vi "Calculadora.vi"() -> ()   [LabVIEW 2019, in "Calculadora.lvlib"]
uses:
  Calculadora.lvlib
panel:
  out "Resultado":dbl
  in  "Borrar":bool
  in  "Division":bool
  in  "Multiplicacion":bool
  in  "Resta":bool
  in  "Numero":dbl
  in  "Suma":bool
  # "CALCULADORA"
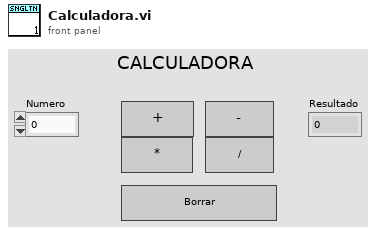
[diagram p1: front panel]
types:
  T1 = typedef "Calculadora.lvlib/Broadcast Events--cluster.ctl" = cluster{"Module Did Init":refnum<user-event>, "Status Updated":refnum<user-event>, "Error Reported":refnum<user-event>, "Did Something":refnum<user-event>, "Module Did Stop":refnum<user-event>, "Update Module Execution Status":refnum<user-event>, "Resultado":refnum<user-event>}
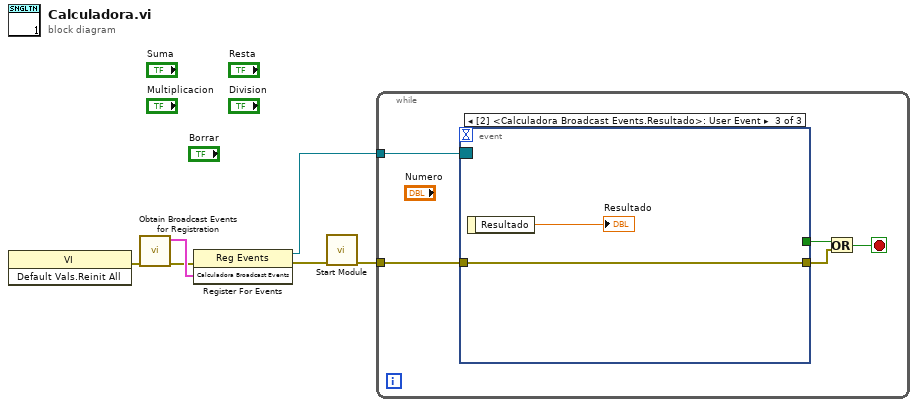
[diagram p0: block diagram]
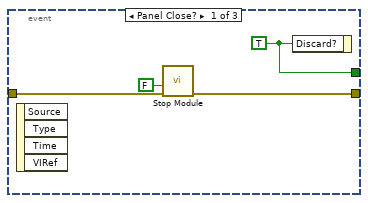
[diagram p2: hidden frame]
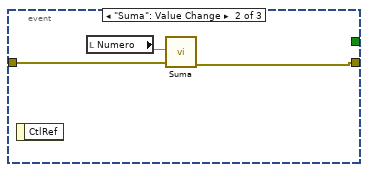
[diagram p3: hidden frame]
diagram:
  n1 = invoke class="VI" method="Default Vals.Reinit All"() -> (error out=w5:errorcluster)  [unwired: 3 in, 2 out]
  n2 = call "Obtain Broadcast Events for Registration.vi"("error in"=w5) -> ("error out"=w4:errorcluster, "Calculadora Broadcast Events"=w6:T1)  [unwired: 8 in, 1 out]
  n3 = register-events(error in=w4, w6) -> (reference out=w2:refnum<event-registration>, error out=w3:errorcluster)  [unwired: 1 in]
  n4 = call "Start Module.vi"("error in"=w3) -> ("error out"=w1:errorcluster)  [unwired: 7 in, 3 out]
  n5 = while {
    tunnel: w2 -> [w11]
    tunnel: w1 -> [w10]
    stop <- w7 stop-if-true
    n6 = event shown="[2] <Calculadora Broadcast Events.Resultado>: User Event" {
      selector: w11 -> [_ _ _]
      dyn-events: _ -> [_ _ _]
      timeout: _ -> [_ _ _]
      tunnel: w10 -> [w15 w18 w19]
      tunnel: [w14 w17 w19] -> w9
      tunnel: [w12 _ _] -> w8
      event Panel Close? {
        w12 = TRUE ("Discard?")
        n7 = event-data() -> ()  [unwired: 1 in, 4 out]
        n8 = call "Stop Module.vi"("error in"=w15, "Wait for Module to Stop? (F)"=FALSE) -> ("error out"=w14:errorcluster)  [unwired: 9 in]
        n9 = event-data("Discard?"=w12) -> ()  [unwired: 1 in, 1 out]
      }
      event "Suma": Value Change {
        n10 = event-data() -> ()  [unwired: 1 in, 1 out]
        n11 = local read "Numero"() -> (w16:dbl)
        n12 = call "Suma.vi"("error in"=w18, "Numero"=w16) -> ("error out"=w17:errorcluster)  [unwired: 9 in]
      }
      event User Event {
        n13 = event-data() -> ("Resultado"=→"Resultado":dbl)  [unwired: 1 in]
      }
    }
    n14 = Or(x=w8, y=w9) -> (x .or. y?=w7:bool)
  }
